vi "XY Graph Select All Plots Event.vi"(8 "Error In":errorcluster, 10 "Select (T)/Deselect":bool=TRUE, 11 "XYGraph Ref":T1) -> (0 "Error Out":errorcluster, 1 "Message":string, 2 "Graph Caption":string, 3 "XYGraph Ref":T1)   [LabVIEW 2019, in "XY Graph Add-Ons.lvlib"]
uses:
  XY Graph Add-Ons.lvlib
  XY Graph Refnum.ctl
  <vilib>/Utility/High Resolution Relative Seconds.vi
panel:
  out "CPU (s)":dbl
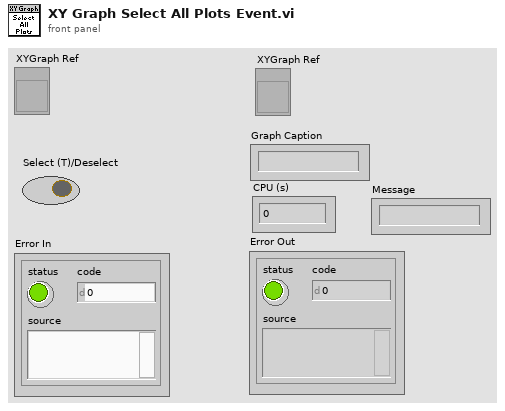
[diagram p1: front panel]
types:
  T1 = typedef "XY Graph Add-Ons.lvlib/XY Graph Refnum.ctl" = refnum<vi>
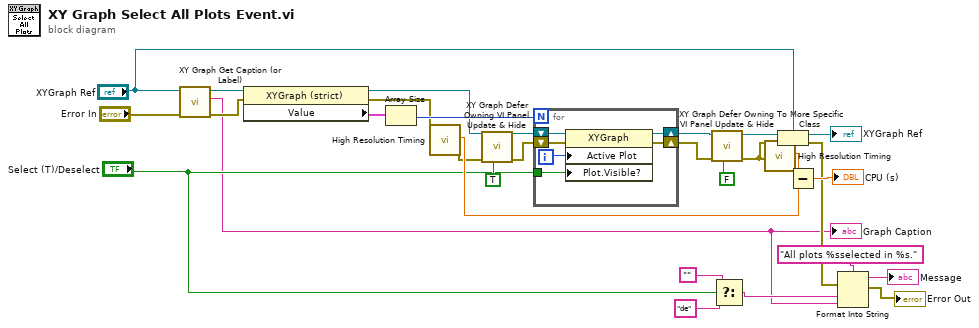
[diagram p0: block diagram]
diagram:
  n1 = call "XY Graph Get Caption (or Label).vi"("error in (no error)"="Error In", "XYGraph in"="XYGraph Ref") -> ("error out"=w2:errorcluster, "Caption (or Label) Text"=w1:string, "XYGraph out"=w4:T1)  [unwired: 7 in]
  "Graph Caption" <- w1
  n2 = property class="XYGraph (strict)"(reference=w4, error in=w2) -> (reference out=w28:T1, error out=w27:errorcluster, "Value"=w30:cluster{"X Array":dbl[], "Y Array":dbl[]}[])
  n3 = Array Size(array=w30) -> (size(s)=w29:i32)
  n4 = call "High Resolution Timing.vi"("Error In"=w27) -> ("elapsed (relative) seconds"=w25:dbl, "Error Out"=w22:errorcluster)  [unwired: 16 in, 1 out]
  n5 = call "XY Graph Defer Owning VI Panel Update & Hide.vi"("Defer Owning Panel Update"=TRUE ("Hide (F)/Show (T) Graph"), "error in (no error)"=w22, "XY Graph Refnum in"=w28) -> ("error out"=w21:errorcluster, "XY Graph Refnum out"=w23:refnum<vi>)  [unwired: 7 in]
  n6 = for {
    N: w29 -> [_]
    shift-right: [w32] -> w20
    shift-left: w23 -> [w36]
    shift-right: [w31] -> w19
    shift-left: w21 -> [w35]
    tunnel: "Select (T)/Deselect" -> [w33]
    i -> [w34]
    n7 = property class="XYGraph"(reference=w36, error in=w35, "Active Plot"=w34, "Plot.Visible?"=w33) -> (reference out=w32:refnum<vi>, error out=w31:errorcluster)
  }
  n8 = call "XY Graph Defer Owning VI Panel Update & Hide.vi"("Defer Owning Panel Update"=FALSE ("Hide (F)/Show (T) Graph"), "error in (no error)"=w19, "XY Graph Refnum in"=w20) -> ("error out"=w16:errorcluster, "XY Graph Refnum out"=w18:refnum<vi>)  [unwired: 7 in]
  n9 = Select(t="", s="Select (T)/Deselect", f="de" ("input 1")) -> (s? t:f=w8:string)
  n10 = call "High Resolution Timing.vi"("Error In"=w16) -> ("elapsed (relative) seconds"=w26:dbl)  [unwired: 16 in, 2 out]
  n11 = To More Specific Class(target class="XYGraph Ref", reference=w18, error in=w16) -> (specific class reference=→"XYGraph Ref":T1, error out=w14:errorcluster)
  n12 = Subtract(x=w26, y=w25) -> (x-y=→"CPU (s)":dbl)
  n13 = Format Into String(format string="All plots %sselected in %s." ("initial string"), error in=w14, w8, w1) -> (resulting string=→"Message":string, error out=→"Error Out":errorcluster)  [unwired: 1 in]
